vi "GeoData.vi"() -> ()   [LabVIEW 2017] (continued)
County\tH1\n81120\t8023\tAntonito\tCO\tCostilla County\tH1\n81152\t8023\tSan luis\tCO\tCostilla County\tH1\n81151\t8023\tSanford\tCO\tCostilla County\tH1\n81126\t8023\tChama\tCO\tCostilla County\tH1\n81133\t8023\tFort garland\tCO\tCostilla County\tH1\n81123\t8023\tBlanca\tCO\tCostilla County\tH1\n81138\t8023\tJaroso\tCO\tCostilla County\tH1\n81039\t8025\tFowler\tCO\tCrowley County\tH1\n81058\t8025\tManzanola\tCO\tCrowley County\tH1\n81076\t8025\tSugar city\tCO\tCrowley County\tH1\n81034\t8025\tOrdway\tCO\tCrowley County\tH1\n81063\t8025\tOrdway\tCO\tCrowley County\tH1\n81062\t8025\tOlney springs\tCO\tCrowley County\tH1\n81033\t8025\tCrowley\tCO\tCrowley County\tH1\n81252\t8027\tWestcliffe\tCO\tCuster County\tH1\n81223\t8027\tCotopaxi\tCO\tCuster County\tH1\n81253\t8027\tWetmore\tCO\tCuster County\tH1\n81226\t8027\tFlorence\tCO\tCuster County\tH1\n81069\t8027\tRye\tCO\tCuster County\tH1\n81410\t8029\tAustin\tCO\tDelta County\tH1\n81418\t8029\tEckert\tCO\tDelta County\tH1\n81420\t8029\tLazear\tCO\tDelta County\tH1\n81428\t8029\tPaonia\tCO\tDelta County\tH1\n81413\t8029\tCedaredge\tCO\tDelta County\tH1\n81419\t8029\tHotchkiss\tCO\tDelta County\tH1\n81415\t8029\tCrawford\tCO\tDelta County\tH1\n81414\t8029\tCory\tCO\tDelta County\tH1\n81434\t8029\tSomerset\tCO\tDelta County\tH1\n81416\t8029\tDelta\tCO\tDelta County\tH1\n80110\t8031\tEnglewood\tCO\tDenver County\tH6\n80224\t8031\tDenver\tCO\tDenver County\tH6\n80218\t8031\tDenver\tCO\tDenver County\tH6\n80247\t8031\tDenver\tCO\tDenver County\tH6\n80266\t8031\tDenver\tCO\tDenver County\tH6\n80290\t8031\tDenver\tCO\tDenver County\tH6\n80293\t8031\tDenver\tCO\tDenver County\tH6\n80259\t8031\tDenver\tCO\tDenver County\tH6\n80221\t8031\tDenver\tCO\tDenver County\tH6\n80246\t8031\tDenver\tCO\tDenver County\tH6\n80208\t8031\tDenver\tCO\tDenver County\tH6\n80014\t8031\tAurora\tCO\tDenver County\tH6\n80127\t8031\tLittleton\tCO\tDenver County\tH6\n80210\t8031\tDenver\tCO\tDenver County\tH6\n80226\t8031\tDenver\tCO\tDenver County\tH6\n80206\t8031\tDenver\tCO\tDenver County\tH6\n80236\t8031\tDenver\tCO\tDenver County\tH6\n80227\t8031\tDenver\tCO\tDenver County\tH6\n80239\t8031\tDenver\tCO\tDenver County\tH6\n80273\t8031\tDenver\tCO\tDenver County\tH6\n80294\t8031\tDenver\tCO\tDenver County\tH6\n80256\t8031\tDenver\tCO\tDenver County\tH6\n80012\t8031\tAurora\tCO\tDenver County\tH6\n80123\t8031\tLittleton\tCO\tDenver County\tH6\n80111\t8031\tEnglewood\tCO\tDenver County\tH6\n80202\t8031\tDenver\tCO\tDenver County\tH6\n80220\t8031\tDenver\tCO\tDenver County\tH6\n80231\t8031\tDenver\tCO\tDenver County\tH6\n80281\t8031\tDenver\tCO\tDenver County\tH6\n80010\t8031\tAurora\tCO\tDenver County\tH6\n80022\t8031\tCommerce city\tCO\tDenver County\tH6\n80219\t8031\tDenver\tCO\tDenver County\tH6\n80222\t8031\tDenver\tCO\tDenver County\tH6\n80212\t8031\tDenver\tCO\tDenver County\tH6\n80217\t8031\tDenver\tCO\tDenver County\tH6\n80264\t8031\tDenver\tCO\tDenver County\tH6\n80211\t8031\tDenver\tCO\tDenver County\tH6\n80207\t8031\tDenver\tCO\tDenver County\tH6\n80214\t8031\tDenver\tCO\tDenver County\tH6\n80223\t8031\tDenver\tCO\tDenver County\tH6\n80230\t8031\tDenver\tCO\tDenver County\tH6\n80238\t8031\tDenver\tCO\tDenver County\tH6\n80263\t8031\tDenver\tCO\tDenver County\tH6\n80257\t8031\tDenver\tCO\tDenver County\tH6\n80274\t8031\tDenver\tCO\tDenver County\tH6\n80243\t8031\tDenver\tCO\tDenver County\tH6\n80271\t8031\tDenver\tCO\tDenver County\tH6\n80033\t8031\tWheat ridge\tCO\tDenver County\tH6\n80204\t8031\tDenver\tCO\tDenver County\tH6\n80203\t8031\tDenver\tCO\tDenver County\tH6\n80249\t8031\tDenver\tCO\tDenver County\tH6\n80299\t8031\tDenver\tCO\tDenver County\tH6\n80250\t8031\tDenver\tCO\tDenver County\tH6\n80248\t8031\tDenver\tCO\tDenver County\tH6\n80265\t8031\tDenver\tCO\tDenver County\tH6\n80261\t8031\tDenver\tCO\tDenver County\tH6\n80201\t8031\tDenver\tCO\tDenver County\tH6\n80216\t8031\tDenver\tCO\tDenver County\tH6\n80205\t8031\tDenver\tCO\tDenver County\tH6\n80209\t8031\tDenver\tCO\tDenver County\tH6\n80232\t8031\tDenver\tCO\tDenver County\tH6\n80235\t8031\tDenver\tCO\tDenver County\tH6\n80237\t8031\tDenver\tCO\tDenver County\tH6\n80291\t8031\tDenver\tCO\tDenver County\tH6\n81324\t8033\tDove creek\tCO\tDolores County\tH1\n81332\t8033\tRico\tCO\tDolores County\tH1\n81320\t8033\tCahone\tCO\tDolores County\tH1\n80104\t8035\tCastle rock\tCO\tDouglas County\tH1\n80108\t8035\tCastle rock\tCO\tDouglas County\tH1\n80163\t8035\tLittleton\tCO\tDouglas County\tH1\n80112\t8035\tEnglewood\tCO\tDouglas County\tH1\n80125\t8035\tLittleton\tCO\tDouglas County\tH1\n80124\t8035\tLone tree\tCO\tDouglas County\tH1\n80129\t8035\tLittleton\tCO\tDouglas County\tH1\n80126\t8035\tLittleton\tCO\tDouglas County\tH1\n80118\t8035\tLarkspur\tCO\tDouglas County\tH1\n80130\t8035\tLittleton\tCO\tDouglas County\tH1\n80109\t8035\tCastle rock\tCO\tDouglas County\tH1\n80138\t8035\tParker\tCO\tDouglas County\tH1\n80131\t8035\tLouviers\tCO\tDouglas County\tH1\n80016\t8035\tAurora\tCO\tDouglas County\tH1\n80106\t8035\tElbert\tCO\tDouglas County\tH1\n80135\t8035\tSedalia\tCO\tDouglas County\tH1\n80433\t8035\tConifer\tCO\tDouglas County\tH1\n80116\t8035\tFranktown\tCO\tDouglas County\tH1\n80134\t8035\tParker\tCO\tDouglas County\tH1\n81645\t8037\tMinturn\tCO\tEagle County\tH1\n81631\t8037\tEagle\tCO\tEagle County\tH1\n81620\t8037\tAvon\tCO\tEagle County\tH1\n81655\t8037\tWolcott\tCO\tEagle County\tH1\n81649\t8037\tRed cliff\tCO\tEagle County\tH1\n80423\t8037\tBond\tCO\tEagle County\tH1\n81657\t8037\tVail\tCO\tEagle County\tH1\n80498\t8037\tSilverthorne\tCO\tEagle County\tH1\n81621\t8037\tBasalt\tCO\tEagle County\tH1\n81637\t8037\tGypsum\tCO\tEagle County\tH1\n81658\t8037\tVail\tCO\tEagle County\tH1\n80463\t8037\tMc coy\tCO\tEagle County\tH1\n81632\t8037\tEdwards\tCO\tEagle County\tH1\n81623\t8037\tCarbondale\tCO\tEagle County\tH1\n81642\t8037\tMeredith\tCO\tEagle County\tH1\n80426\t8037\tBurns\tCO\tEagle County\tH1\n80832\t8039\tRamah\tCO\tElbert County\tH1\n80105\t8039\tDeer trail\tCO\tElbert County\tH1\n80102\t8039\tBennett\tCO\tElbert County\tH1\n80107\t8039\tElizabeth\tCO\tElbert County\tH1\n80117\t8039\tKiowa\tCO\tElbert County\tH1\n80138\t8039\tParker\tCO\tElbert County\tH1\n80808\t8039\tCalhan\tCO\tElbert County\tH1\n80831\t8039\tPeyton\tCO\tElbert County\tH1\n80101\t8039\tAgate\tCO\tElbert County\tH1\n80106\t8039\tElbert\tCO\tElbert County\tH1\n80116\t8039\tFranktown\tCO\tElbert County\tH1\n80134\t8039\tParker\tCO\tElbert County\tH1\n80833\t8039\tRush\tCO\tElbert County\tH1\n80835\t8039\tSimla\tCO\tElbert County\tH1\n80828\t8039\tLimon\tCO\tElbert County\tH1\n80830\t8039\tMatheson\tCO\tElbert County\tH1\n80903\t8041\tColorado springs\tCO\tEl Paso County\tH1\n80949\t8041\tColorado springs\tCO\tEl Paso County\tH1\n80932\t8041\tColorado springs\tCO\tEl Paso County\tH1\n80901\t8041\tColorado springs\tCO\tEl Paso County\tH1\n80819\t8041\tGreen mountain falls\tCO\tEl Paso County\tH1\n80941\t8041\tColorado springs\tCO\tEl Paso County\tH1\n80917\t8041\tColorado springs\tCO\tEl Paso County\tH1\n80923\t8041\tColorado springs\tCO\tEl Paso County\tH1\n80928\t8041\tColorado springs\tCO\tEl Paso County\tH1\n80933\t8041\tColorado springs\tCO\tEl Paso County\tH1\n80832\t8041\tRamah\tCO\tEl Paso County\tH1\n80938\t8041\tColorado springs\tCO\tEl Paso County\tH1\n80132\t8041\tMonument\tCO\tEl Paso County\tH1\n80921\t8041\tColorado springs\tCO\tEl Paso County\tH1\n80926\t8041\tColorado springs\tCO\tEl Paso County\tH1\n80906\t8041\tColorado springs\tCO\tEl Paso County\tH1\n80907\t8041\tColorado springs\tCO\tEl Paso County\tH1\n80913\t8041\tColorado springs\tCO\tEl Paso County\tH1\n80809\t8041\tCascade\tCO\tEl Paso County\tH1\n80929\t8041\tColorado springs\tCO\tEl Paso County\tH1\n80935\t8041\tColorado springs\tCO\tEl Paso County\tH1\n80841\t8041\tUsaf academy\tCO\tEl Paso County\tH1\n80931\t8041\tColorado springs\tCO\tEl Paso County\tH1\n80942\t8041\tColorado springs\tCO\tEl Paso County\tH1\n80817\t8041\tFountain\tCO\tEl Paso County\tH1\n80920\t8041\tColorado springs\tCO\tEl Paso County\tH1\n80915\t8041\tColorado springs\tCO\tEl Paso County\tH1\n80936\t8041\tColorado springs\tCO\tEl Paso County\tH1\n81008\t8041\tPueblo\tCO\tEl Paso County\tH1\n80133\t8041\tPalmer lake\tCO\tEl Paso County\tH1\n80930\t8041\tColorado springs\tCO\tEl Paso County\tH1\n80977\t8041\tColorado springs\tCO\tEl Paso County\tH1\n80808\t8041\tCalhan\tCO\tEl Paso County\tH1\n80831\t8041\tPeyton\tCO\tEl Paso County\tH1\n80829\t8041\tManitou springs\tCO\tEl Paso County\tH1\n80911\t8041\tColorado springs\tCO\tEl Paso County\tH1\n80908\t8041\tColorado springs\tCO\tEl Paso County\tH1\n80927\t8041\tColorado springs\tCO\tEl Paso County\tH1\n80904\t8041\tColorado springs\tCO\tEl Paso County\tH1\n80924\t8041\tColorado springs\tCO\tEl Paso County\tH1\n80939\t8041\tColorado springs\tCO\tEl Paso County\tH1\n80962\t8041\tColorado springs\tCO\tEl Paso County\tH1\n80934\t8041\tColorado springs\tCO\tEl Paso County\tH1\n80950\t8041\tColorado springs\tCO\tEl Paso County\tH1\n80106\t8041\tElbert\tCO\tEl Paso County\tH1\n80914\t8041\tColorado springs\tCO\tEl Paso County\tH1\n80918\t8041\tColorado springs\tCO\tEl Paso County\tH1\n80919\t8041\tColorado springs\tCO\tEl Paso County\tH1\n80916\t8041\tColorado springs\tCO\tEl Paso County\tH1\n80947\t8041\tColorado springs\tCO\tEl Paso County\tH1\n80946\t8041\tColorado springs\tCO\tEl Paso County\tH1\n80833\t8041\tRush\tCO\tEl Paso County\tH1\n80910\t8041\tColorado springs\tCO\tEl Paso County\tH1\n80909\t8041\tColorado springs\tCO\tEl Paso County\tH1\n80905\t8041\tColorado springs\tCO\tEl Paso County\tH1\n80951\t8041\tColorado springs\tCO\tEl Paso County\tH1\n80840\t8041\tUsaf academy\tCO\tEl Paso County\tH1\n80864\t8041\tYoder\tCO\tEl Paso County\tH1\n80835\t8041\tSimla\tCO\tEl Paso County\tH1\n80912\t8041\tColorado springs\tCO\tEl Paso County\tH1\n80863\t8041\tWoodland park\tCO\tEl Paso County\tH1\n80922\t8041\tColorado springs\tCO\tEl Paso County\tH1\n80902\t8041\tColorado springs\tCO\tEl Paso County\tH1\n80925\t8041\tColorado springs\tCO\tEl Paso County\tH1\n80960\t8041\tColorado springs\tCO\tEl Paso County\tH1\n80970\t8041\tColorado springs\tCO\tEl Paso County\tH1\n80937\t8041\tColorado springs\tCO\tEl Paso County\tH1\n80997\t8041\tColorado springs\tCO\tEl Paso County\tH1\n81240\t8043\tPenrose\tCO\tFremont County\tH1\n81221\t8043\tCoal creek\tCO\tFremont County\tH1\n81232\t8043\tHillside\tCO\tFremont County\tH1\n81252\t8043\tWestcliffe\tCO\tFremont County\tH1\n80926\t8043\tColorado springs\tCO\tFremont County\tH1\n81244\t8043\tRockvale\tCO\tFremont County\tH1\n81212\t8043\tCanon city\tCO\tFremont County\tH1\n81223\t8043\tCotopaxi\tCO\tFremont County\tH1\n81233\t8043\tHoward\tCO\tFremont County\tH1\n81222\t8043\tCoaldale\tCO\tFremont County\tH1\n81290\t8043\tFlorence\tCO\tFremont County\tH1\n81201\t8043\tSalida\tCO\tFremont County\tH1\n81253\t8043\tWetmore\tCO\tFremont County\tH1\n81226\t8043\tFlorence\tCO\tFremont County\tH1\n81215\t8043\tCanon city\tCO\tFremont County\tH1\n80816\t8043\tFlorissant\tCO\tFremont County\tH1\n81641\t8045\tMeeker\tCO\tGarfield County\tH1\n81652\t8045\tSilt\tCO\tGarfield County\tH1\n81647\t8045\tNew castle\tCO\tGarfield County\tH1\n81602\t8045\tGlenwood springs\tCO\tGarfield County\tH1\n81635\t8045\tParachute\tCO\tGarfield County\tH1\n81630\t8045\tDe beque\tCO\tGarfield County\tH1\n81637\t8045\tGypsum\tCO\tGarfield County\tH1\n81601\t8045\tGlenwood springs\tCO\tGarfield County\tH1\n81623\t8045\tCarbondale\tCO\tGarfield County\tH1\n81650\t8045\tRifle\tCO\tGarfield County\tH1\n80422\t8047\tBlack hawk\tCO\tGilpin County\tH1\n80474\t8047\tRollinsville\tCO\tGilpin County\tH1\n80427\t8047\tCentral city\tCO\tGilpin County\tH1\n80403\t8047\tGolden\tCO\tGilpin County\tH1\n80446\t8049\tGranby\tCO\tGrand County\tH1\n80447\t8049\tGrand lake\tCO\tGrand County\tH1\n80442\t8049\tFraser\tCO\tGrand County\tH1\n80482\t8049\tWinter park\tCO\tGrand County\tH1\n80423\t8049\tBond\tCO\tGrand County\tH1\n80498\t8049\tSilverthorne\tCO\tGrand County\tH1\n80459\t8049\tKremmling\tCO\tGrand County\tH1\n80478\t8049\tTabernash\tCO\tGrand County\tH1\n80451\t8049\tHot sulphur springs\tCO\tGrand County\tH1\n80468\t8049\tParshall\tCO\tGrand County\tH1\n81225\t8051\tCrested butte\tCO\tGunnison County\tH1\n81241\t8051\tPitkin\tCO\tGunnison County\tH1\n81428\t8051\tPaonia\tCO\tGunnison County\tH1\n81239\t8051\tParlin\tCO\tGunnison County\tH1\n81230\t8051\tGunnison\tCO\tGunnison County\tH1\n81220\t8051\tCimarron\tCO\tGunnison County\tH1\n81237\t8051\tOhio city\tCO\tGunnison County\tH1\n81210\t8051\tAlmont\tCO\tGunnison County\tH1\n81243\t8051\tPowderhorn\tCO\tGunnison County\tH1\n81434\t8051\tSomerset\tCO\tGunnison County\tH1\n81231\t8051\tGunnison\tCO\tGunnison County\tH1\n81623\t8051\tCarbondale\tCO\tGunnison County\tH1\n81224\t8051\tCrested butte\tCO\tGunnison County\tH1\n81235\t8053\tLake city\tCO\tHinsdale County\tH1\n81147\t8053\tPagosa springs\tCO\tHinsdale County\tH1\n81130\t8053\tCreede\tCO\tHinsdale County\tH1\n81040\t8055\tGardner\tCO\tHuerfano County\tH1\n81089\t8055\tWalsenburg\tCO\tHuerfano County\tH1\n81055\t8055\tLa veta\tCO\tHuerfano County\tH1\n81069\t8055\tRye\tCO\tHuerfano County\tH1\n80430\t8057\tCoalmont\tCO\tJackson County\tH1\n80473\t8057\tRand\tCO\tJackson County\tH1\n80434\t8057\tCowdrey\tCO\tJackson County\tH1\n80480\t8057\tWalden\tCO\tJackson County\tH1\n80439\t8059\tEvergreen\tCO\tJefferson County\tH1\n80454\t8059\tIndian hills\tCO\tJefferson County\tH1\n80004\t8059\tArvada\tCO\tJefferson County\tH1\n80215\t8059\tDenver\tCO\tJefferson County\tH1\n80228\t8059\tDenver\tCO\tJefferson County\tH1\n80401\t8059\tGolden\tCO\tJefferson County\tH1\n80002\t8059\tArvada\tCO\tJefferson County\tH1\n80127\t8059\tLittleton\tCO\tJefferson County\tH1\n80125\t8059\tLittleton\tCO\tJefferson County\tH1\n80226\t8059\tDenver\tCO\tJefferson County\tH1\n80227\t8059\tDenver\tCO\tJefferson County\tH1\n80303\t8059\tBoulder\tCO\tJefferson County\tH1\n80465\t8059\tMorrison\tCO\tJefferson County\tH1\n80162\t8059\tLittleton\tCO\tJefferson County\tH1\n80453\t8059\tIdledale\tCO\tJefferson County\tH1\n80123\t8059\tLittleton\tCO\tJefferson County\tH1\n80437\t8059\tEvergreen\tCO\tJefferson County\tH1\n80006\t8059\tArvada\tCO\tJefferson County\tH1\n80001\t8059\tArvada\tCO\tJefferson County\tH1\n80419\t8059\tGolden\tCO\tJefferson County\tH1\n80003\t8059\tArvada\tCO\tJefferson County\tH1\n80020\t8059\tBroomfield\tCO\tJefferson County\tH1\n80007\t8059\tArvada\tCO\tJefferson County\tH1\n80212\t8059\tDenver\tCO\tJefferson County\tH1\n80021\t8059\tBroomfield\tCO\tJefferson County\tH1\n80031\t8059\tWestminster\tCO\tJefferson County\tH1\n80135\t8059\tSedalia\tCO\tJefferson County\tH1\n80214\t8059\tDenver\tCO\tJefferson County\tH1\n80403\t8059\tGolden\tCO\tJefferson County\tH1\n80433\t8059\tConifer\tCO\tJefferson County\tH1\n80402\t8059\tGolden\tCO\tJefferson County\tH1\n80034\t8059\tWheat ridge\tCO\tJefferson County\tH1\n80457\t8059\tKittredge\tCO\tJefferson County\tH1\n80033\t8059\tWheat ridge\tCO\tJefferson County\tH1\n80128\t8059\tLittleton\tCO\tJefferson County\tH1\n80204\t8059\tDenver\tCO\tJefferson County\tH1\n80421\t8059\tBailey\tCO\tJefferson County\tH1\n80225\t8059\tDenver\tCO\tJefferson County\tH1\n80425\t8059\tBuffalo creek\tCO\tJefferson County\tH1\n80005\t8059\tArvada\tCO\tJefferson County\tH1\n80232\t8059\tDenver\tCO\tJefferson County\tH1\n80235\t8059\tDenver\tCO\tJefferson County\tH1\n80470\t8059\tPine\tCO\tJefferson County\tH1\n81045\t8061\tHaswell\tCO\tKiowa County\tH1\n81092\t8061\tWiley\tCO\tKiowa County\tH1\n81036\t8061\tEads\tCO\tKiowa County\tH1\n81047\t8061\tHolly\tCO\tKiowa County\tH1\n81071\t8061\tSheridan lake\tCO\tKiowa County\tH1\n81021\t8061\tArlington\tCO\tKiowa County\tH1\n80834\t8063\tSeibert\tCO\tKit Carson County\tH1\n80861\t8063\tVona\tCO\tKit Carson County\tH1\n80805\t8063\tBethune\tCO\tKit Carson County\tH1\n80836\t8063\tStratton\tCO\tKit Carson County\tH1\n80807\t8063\tBurlington\tCO\tKit Carson County\tH1\n80815\t8063\tFlagler\tCO\tKit Carson County\tH1\n80461\t8065\tLeadville\tCO\tLake County\tH1\n81251\t8065\tTwin lakes\tCO\tLake County\tH1\n80429\t8065\tClimax\tCO\tLake County\tH1\n81228\t8065\tGranite\tCO\tLake County\tH1\n81326\t8067\tHesperus\tCO\tLa Plata County\tH1\n81137\t8067\tIgnacio\tCO\tLa Plata County\tH1\n81303\t8067\tDurango\tCO\tLa Plata County\tH1\n81302\t8067\tDurango\tCO\tLa Plata County\tH1\n81329\t8067\tMarvel\tCO\tLa Plata County\tH1\n81301\t8067\tDurango\tCO\tLa Plata County\tH1\n81122\t8067\tBayfield\tCO\tLa Plata County\tH1\n81328\t8067\tMancos\tCO\tLa Plata County\tH1\n80549\t8069\tWellington\tCO\tLarimer County\tH1\n80547\t8069\tTimnath\tCO\tLarimer County\tH1\n80525\t8069\tFort collins\tCO\tLarimer County\tH1\n80538\t8069\tLoveland\tCO\tLarimer County\tH1\n80537\t8069\tLoveland\tCO\tLarimer County\tH1\n80553\t8069\tFort collins\tCO\tLarimer County\tH1\n80513\t8069\tBerthoud\tCO\tLarimer County\tH1\n80517\t8069\tEstes park\tCO\tLarimer County\tH1\n80521\t8069\tFort collins\tCO\tLarimer County\tH1\n80430\t8069\tCoalmont\tCO\tLarimer County\tH1\n80512\t8069\tBellvue\tCO\tLarimer County\tH1\n80510\t8069\tAllenspark\tCO\tLarimer County\tH1\n80532\t8069\tGlen haven\tCO\tLarimer County\tH1\n80511\t8069\tEstes park\tCO\tLarimer County\tH1\n80535\t8069\tLaporte\tCO\tLarimer County\tH1\n80527\t8069\tFort collins\tCO\tLarimer County\tH1\n80503\t8069\tLongmont\tCO\tLarimer County\tH1\n80541\t8069\tMasonville\tCO\tLarimer County\tH1\n80528\t8069\tFort collins\tCO\tLarimer County\tH1\n80534\t8069\tJohnstown\tCO\tLarimer County\tH1\n80545\t8069\tRed feather lakes\tCO\tLarimer County\tH1\n80524\t8069\tFort collins\tCO\tLarimer County\tH1\n80536\t8069\tLivermore\tCO\tLarimer County\tH1\n80522\t8069\tFort collins\tCO\tLarimer County\tH1\n80526\t8069\tFort collins\tCO\tLarimer County\tH1\n80550\t8069\tWindsor\tCO\tLarimer County\tH1\n80504\t8069\tLongmont\tCO\tLarimer County\tH1\n80515\t8069\tDrake\tCO\tLarimer County\tH1\n80612\t8069\tCarr\tCO\tLarimer County\tH1\n80540\t8069\tLyons\tCO\tLarimer County\tH1\n80523\t8069\tFort collins\tCO\tLarimer County\tH1\n80539\t8069\tLoveland\tCO\tLarimer County\tH1\n81039\t8071\tFowler\tCO\tLas Animas County\tH1\n81046\t8071\tHoehne\tCO\tLas Animas County\tH1\n81089\t8071\tWalsenburg\tCO\tLas Animas County\tH1\n81020\t8071\tAguilar\tCO\tLas Animas County\tH1\n81081\t8071\tTrinchera\tCO\tLas Animas County\tH1\n81091\t8071\tWeston\tCO\tLas Animas County\tH1\n81024\t8071\tBoncarbo\tCO\tLas Animas County\tH1\n81082\t8071\tTrinidad\tCO\tLas Animas County\tH1\n81049\t8071\tKim\tCO\tLas Animas County\tH1\n81027\t8071\tBranson\tCO\tLas Animas County\tH1\n81054\t8071\tLas animas\tCO\tLas Animas County\tH1\n81059\t8071\tModel\tCO\tLas Animas County\tH1\n81064\t8071\tPritchett\tCO\tLas Animas County\tH1\n81076\t8073\tSugar city\tCO\tLincoln County\tH1\n80826\t8073\tLimon\tCO\tLincoln County\tH1\n80832\t8073\tRamah\tCO\tLincoln County\tH1\n81045\t8073\tHaswell\tCO\tLincoln County\tH1\n80821\t8073\tHugo\tCO\tLincoln County\tH1\n81063\t8073\tOrdway\tCO\tLincoln County\tH1\n80804\t8073\tArriba\tCO\tLincoln County\tH1\n80833\t8073\tRush\tCO\tLincoln County\tH1\n80815\t8073\tFlagler\tCO\tLincoln County\tH1\n81021\t8073\tArlington\tCO\tLincoln County\tH1\n80828\t8073\tLimon\tCO\tLincoln County\tH1\n80823\t8073\tKarval\tCO\tLincoln County\tH1\n80818\t8073\tGenoa\tCO\tLincoln County\tH1\n80741\t8075\tMerino\tCO\tLogan County\tH1\n80726\t8075\tCrook\tCO\tLogan County\tH1\n80751\t8075\tSterling\tCO\tLogan County\tH1\n80731\t8075\tHaxtun\tCO\tLogan County\tH1\n80747\t8075\tPeetz\tCO\tLogan County\tH1\n80745\t8075\tPadroni\tCO\tLogan County\tH1\n80736\t8075\tIliff\tCO\tLogan County\tH1\n80728\t8075\tFleming\tCO\tLogan County\tH1\n80722\t8075\tAtwood\tCO\tLogan County\tH1\n81523\t8077\tGlade park\tCO\tMesa County\tH1\n81504\t8077\tGrand junction\tCO\tMesa County\tH1\n81521\t8077\tFruita\tCO\tMesa County\tH1\n81507\t8077\tGrand junction\tCO\tMesa County\tH1\n81502\t8077\tGrand junction\tCO\tMesa County\tH1\n81635\t8077\tParachute\tCO\tMesa County\tH1\n81520\t8077\tClifton\tCO\tMesa County\tH1\n81505\t8077\tGrand junction\tCO\tMesa County\tH1\n81524\t8077\tLoma\tCO\tMesa County\tH1\n81501\t8077\tGrand junction\tCO\tMesa County\tH1\n81527\t8077\tWhitewater\tCO\tMesa County\tH1\n81525\t8077\tMack\tCO\tMesa County\tH1\n81630\t8077\tDe beque\tCO\tMesa County\tH1\n81522\t8077\tGateway\tCO\tMesa County\tH1\n81503\t8077\tGrand junction\tCO\tMesa County\tH1\n81506\t8077\tGrand junction\tCO\tMesa County\tH1\n81646\t8077\tMolina\tCO\tMesa County\tH1\n81526\t8077\tPalisade\tCO\tMesa County\tH1\n81624\t8077\tCollbran\tCO\tMesa County\tH1\n81643\t8077\tMesa\tCO\tMesa County\tH1\n81154\t8079\tSouth fork\tCO\tMineral County\tH1\n81130\t8079\tCreede\tCO\tMineral County\tH1\n81638\t8081\tHamilton\tCO\tMoffat County\tH1\n81641\t8081\tMeeker\tCO\tMoffat County\tH1\n81610\t8081\tDinosaur\tCO\tMoffat County\tH1\n81653\t8081\tSlater\tCO\tMoffat County\tH1\n81633\t8081\tDinosaur\tCO\tMoffat County\tH1\n81640\t8081\tMaybell\tCO\tMoffat County\tH1\n81625\t8081\tCraig\tCO\tMoffat County\tH1\n81335\t8083\tYellow jacket\tCO\tMontezuma County\tH1\n81330\t8083\tMesa verde national park\tCO\tMontezuma County\tH1\n81323\t8083\tDolores\tCO\tMontezuma County\tH1\n81321\t8083\tCortez\tCO\tMontezuma County\tH1\n81328\t8083\tMancos\tCO\tMontezuma County\tH1\n81327\t8083\tLewis\tCO\tMontezuma County\tH1\n81331\t8083\tPleasant view\tCO\tMontezuma County\tH1\n81334\t8083\tTowaoc\tCO\tMontezuma County\tH1\n81402\t8085\tMontrose\tCO\tMontrose County\tH1\n81424\t8085\tNucla\tCO\tMontrose County\tH1\n81220\t8085\tCimarron\tCO\tMontrose County\tH1\n81429\t8085\tParadox\tCO\tMontrose County\tH1\n81403\t8085\tMontrose\tCO\tMontrose County\tH1\n81425\t8085\tOlathe\tCO\tMontrose County\tH1\n81415\t8085\tCrawford\tCO\tMontrose County\tH1\n81401\t8085\tMontrose\tCO\tMontrose County\tH1\n81411\t8085\tBedrock\tCO\tMontrose County\tH1\n81416\t8085\tDelta\tCO\tMontrose County\tH1\n81431\t8085\tRedvale\tCO\tMontrose County\tH1\n81422\t8085\tNaturita\tCO\tMontrose County\tH1\n80701\t8087\tFort morgan\tCO\tMorgan County\tH1\n80654\t8087\tWiggins\tCO\tMorgan County\tH1\n80741\t8087\tMerino\tCO\tMorgan County\tH1\n80653\t8087\tWeldona\tCO\tMorgan County\tH1\n80705\t8087\tLog lane village\tCO\tMorgan County\tH1\n80754\t8087\tStoneham\tCO\tMorgan County\tH1\n80649\t8087\tOrchard\tCO\tMorgan County\tH1\n80733\t8087\tHillrose\tCO\tMorgan County\tH1\n80750\t8087\tSnyder\tCO\tMorgan County\tH1\n80723\t8087\tBrush\tCO\tMorgan County\tH1\n80742\t8087\tNew raymer\tCO\tMorgan County\tH1\n81039\t8089\tFowler\tCO\tOtero County\tH1\n81058\t8089\tManzanola\tCO\tOtero County\tH1\n81050\t8089\tLa junta\tCO\tOtero County\tH1\n81030\t8089\tCheraw\tCO\tOtero County\tH1\n81067\t8089\tRocky ford\tCO\tOtero County\tH1\n81024\t8089\tBoncarbo\tCO\tOtero County\tH1\n81082\t8089\tTrinidad\tCO\tOtero County\tH1\n81077\t8089\tSwink\tCO\tOtero County\tH1\n81059\t8089\tModel\tCO\tOtero County\tH1\n81432\t8091\tRidgway\tCO\tOuray County\tH1\n81403\t8091\tMontrose\tCO\tOuray County\tH1\n81427\t8091\tOuray\tCO\tOuray County\tH1\n80827\t8093\tLake george\tCO\tPark County\tH1\n80420\t8093\tAlma\tCO\tPark County\tH1\n80432\t8093\tComo\tCO\tPark County\tH1\n80475\t8093\tShawnee\tCO\tPark County\tH1\n80448\t8093\tGrant\tCO\tPark County\tH1\n80456\t8093\tJefferson\tCO\tPark County\tH1\n80440\t8093\tFairplay\tCO\tPark County\tH1\n80421\t8093\tBailey\tCO\tPark County\tH1\n80816\t8093\tFlorissant\tCO\tPark County\tH1\n80820\t8093\tGuffey\tCO\tPark County\tH1\n80470\t8093\tPine\tCO\tPark County\tH1\n80449\t8093\tHartsel\tCO\tPark County\tH1\n80731\t8095\tHaxtun\tCO\tPhillips County\tH1\n80721\t8095\tAmherst\tCO\tPhillips County\tH1\n80734\t8095\tHolyoke\tCO\tPhillips County\tH1\n80744\t8095\tOvid\tCO\tPhillips County\tH1\n80746\t8095\tPaoli\tCO\tPhillips County\tH1\n81654\t8097\tSnowmass\tCO\tPitkin County\tH1\n81611\t8097\tAspen\tCO\tPitkin County\tH1\n81615\t8097\tSnowmass village\tCO\tPitkin County\tH1\n81621\t8097\tBasalt\tCO\tPitkin County\tH1\n81656\t8097\tWoody creek\tCO\tPitkin County\tH1\n81612\t8097\tAspen\tCO\tPitkin County\tH1\n81623\t8097\tCarbondale\tCO\tPitkin County\tH1\n81642\t8097\tMeredith\tCO\tPitkin County\tH1\n81052\t8099\tLamar\tCO\tProwers County\tH1\n81092\t8099\tWiley\tCO\tProwers County\tH1\n81043\t8099\tHartman\tCO\tProwers County\tH1\n81090\t8099\tWalsh\tCO\tProwers County\tH1\n81047\t8099\tHolly\tCO\tProwers County\tH1\n81041\t8099\tGranada\tCO\tProwers County\tH1\n81039\t8101\tFowler\tCO\tPueblo County\tH1\n81002\t8101\tPueblo\tCO\tPueblo County\tH1\n81010\t8101\tPueblo\tCO\tPueblo County\tH1\n81007\t8101\tPueblo\tCO\tPueblo County\tH1\n81009\t8101\tPueblo\tCO\tPueblo County\tH1\n80817\t8101\tFountain\tCO\tPueblo County\tH1\n81004\t8101\tPueblo\tCO\tPueblo County\tH1\n81008\t8101\tPueblo\tCO\tPueblo County\tH1\n81025\t8101\tBoone\tCO\tPueblo County\tH1\n81062\t8101\tOlney springs\tCO\tPueblo County\tH1\n81001\t8101\tPueblo\tCO\tPueblo County\tH1\n81023\t8101\tBeulah\tCO\tPueblo County\tH1\n81253\t8101\tWetmore\tCO\tPueblo County\tH1\n81006\t8101\tPueblo\tCO\tPueblo County\tH1\n81011\t8101\tPueblo\tCO\tPueblo County\tH1\n81012\t8101\tPueblo\tCO\tPueblo County\tH1\n81022\t8101\tAvondale\tCO\tPueblo County\tH1\n81069\t8101\tRye\tCO\tPueblo County\tH1\n81005\t8101\tPueblo\tCO\tPueblo County\tH1\n81003\t8101\tPueblo\tCO\tPueblo County\tH1\n81019\t8101\tColorado city\tCO\tPueblo County\tH1\n81638\t8103\tHamilton\tCO\tRio Blanco County\tH1\n81641\t8103\tMeeker\tCO\tRio Blanco County\tH1\n81648\t8103\tRangely\tCO\tRio Blanco County\tH1\n81650\t8103\tRifle\tCO\tRio Blanco County\tH1\n81135\t8105\tHomelake\tCO\tRio Grande County\tH1\n81101\t8105\tAlamosa\tCO\tRio Grande County\tH1\n81132\t8105\tDel norte\tCO\tRio Grande County\tH1\n81125\t8105\tCenter\tCO\tRio Grande County\tH1\n81140\t8105\tLa jara\tCO\tRio Grande County\tH1\n81154\t8105\tSouth fork\tCO\tRio Grande County\tH1\n81144\t8105\tMonte vista\tCO\tRio Grande County\tH1\n81638\t8107\tHamilton\tCO\tRoutt County\tH1\n80483\t8107\tYampa\tCO\tRoutt County\tH1\n80467\t8107\tOak creek\tCO\tRoutt County\tH1\n81639\t8107\tHayden\tCO\tRoutt County\tH1\n80479\t8107\tToponas\tCO\tRoutt County\tH1\n80469\t8107\tPhippsburg\tCO\tRoutt County\tH1\n80487\t8107\tSteamboat springs\tCO\tRoutt County\tH1\n80463\t8107\tMc coy\tCO\tRoutt County\tH1\n80477\t8107\tSteamboat springs\tCO\tRoutt County\tH1\n80428\t8107\tClark\tCO\tRoutt County\tH1\n81155\t8109\tVilla grove\tCO\tSaguache County\tH1\n81149\t8109\tSaguache\tCO\tSaguache County\tH1\n81230\t8109\tGunnison\tCO\tSaguache County\tH1\n81143\t8109\tMoffat\tCO\tSaguache County\tH1\n81132\t8109\tDel norte\tCO\tSaguache County\tH1\n81248\t8109\tSargents\tCO\tSaguache County\tH1\n81125\t8109\tCenter\tCO\tSaguache County\tH1\n81136\t8109\tHooper\tCO\tSaguache County\tH1\n81131\t8109\tCrestone\tCO\tSaguache County\tH1\n81432\t8111\tRidgway\tCO\tSan Juan County\tH1\n81301\t8111\tDurango\tCO\tSan Juan County\tH1\n81433\t8111\tSilverton\tCO\tSan Juan County\tH1\n81435\t8113\tTelluride\tCO\tSan Miguel County\tH1\n81432\t8113\tRidgway\tCO\tSan Miguel County\tH1\n81426\t8113\tOphir\tCO\tSan Miguel County\tH1\n81423\t8113\tNorwood\tCO\tSan Miguel County\tH1\n81325\t8113\tEgnar\tCO\tSan Miguel County\tH1\n81430\t8113\tPlacerville\tCO\tSan Miguel County\tH1\n80721\t8115\tAmherst\tCO\tSedgwick County\tH1\n80737\t8115\tJulesburg\tCO\tSedgwick County\tH1\n80749\t8115\tSedgwick\tCO\tSedgwick County\tH1\n80744\t8115\tOvid\tCO\tSedgwick County\tH1\n80443\t8117\tFrisco\tCO\tSummit County\tH1\n80424\t8117\tBreckenridge\tCO\tSummit County\tH1\n80435\t8117\tDillon\tCO\tSummit County\tH1\n80497\t8117\tSilverthorne\tCO\tSummit County\tH1\n80498\t8117\tSilverthorne\tCO\tSummit County\tH1\n80813\t8119\tCripple creek\tCO\tTeller County\tH1\n80827\t8119\tLake george\tCO\tTeller County\tH1\n80814\t8119\tDivide\tCO\tTeller County\tH1\n80906\t8119\tColorado springs\tCO\tTeller County\tH1\n80866\t8119\tWoodland park\tCO\tTeller County\tH1\n80860\t8119\tVictor\tCO\tTeller County\tH1\n80135\t8119\tSedalia\tCO\tTeller County\tH1\n80816\t8119\tFlorissant\tCO\tTeller County\tH1\n80863\t8119\tWoodland park\tCO\tTeller County\tH1\n80741\t8121\tMerino\tCO\tWashington County\tH1\n80834\t8121\tSeibert\tCO\tWashington County\tH1\n80759\t8121\tYuma\tCO\tWashington County\tH1\n80743\t8121\tOtis\tCO\tWashington County\tH1\n80812\t8121\tCope\tCO\tWashington County\tH1\n80801\t8121\tAnton\tCO\tWashington County\tH1\n80733\t8121\tHillrose\tCO\tWashington County\tH1\n80757\t8121\tWoodrow\tCO\tWashington County\tH1\n80723\t8121\tBrush\tCO\tWashington County\tH1\n80720\t8121\tAkron\tCO\tWashington County\tH1\n80818\t8121\tGenoa\tCO\tWashington County\tH1\n80740\t8121\tLindon\tCO\tWashington County\tH1\n80642\t8123\tHudson\tCO\tWeld County\tH1\n80549\t8123\tWellington\tCO\tWeld County\tH1\n80654\t8123\tWiggins\tCO\tWeld County\tH1\n80729\t8123\tGrover\tCO\tWeld County\tH1\n80741\t8123\tMerino\tCO\tWeld County\tH1\n80520\t8123\tFirestone\tCO\tWeld County\tH1\n80646\t8123\tLucerne\tCO\tWeld County\tH1\n80537\t8123\tLoveland\tCO\tWeld County\tH1\n80732\t8123\tHereford\tCO\tWeld County\tH1\n80615\t8123\tEaton\tCO\tWeld County\tH1\n80513\t8123\tBerthoud\tCO\tWeld County\tH1\n80645\t8123\tLa salle\tCO\tWeld County\tH1\n80648\t8123\tNunn\tCO\tWeld County\tH1\n80754\t8123\tStoneham\tCO\tWeld County\tH1\n80634\t8123\tGreeley\tCO\tWeld County\tH1\n80644\t8123\tKersey\tCO\tWeld County\tH1\n80632\t8123\tGreeley\tCO\tWeld County\tH1\n80543\t8123\tMilliken\tCO\tWeld County\tH1\n80516\t8123\tErie\tCO\tWeld County\tH1\n80649\t8123\tOrchard\tCO\tWeld County\tH1\n80624\t8123\tGill\tCO\tWeld County\tH1\n80620\t8123\tEvans\tCO\tWeld County\tH1\n80745\t8123\tPadroni\tCO\tWeld County\tH1\n80611\t8123\tBriggsdale\tCO\tWeld County\tH1\n80633\t8123\tGreeley\tCO\tWeld County\tH1\n80631\t8123\tGreeley\tCO\tWeld County\tH1\n80534\t8123\tJohnstown\tCO\tWeld County\tH1\n80621\t8123\tFort lupton\tCO\tWeld County\tH1\n80643\t8123\tKeenesburg\tCO\tWeld County\tH1\n80524\t8123\tFort collins\tCO\tWeld County\tH1\n80542\t8123\tMead\tCO\tWeld County\tH1\n80651\t8123\tPlatteville\tCO\tWeld County\tH1\n80639\t8123\tGreeley\tCO\tWeld County\tH1\n80652\t8123\tRoggen\tCO\tWeld County\tH1\n80550\t8123\tWindsor\tCO\tWeld County\tH1\n80504\t8123\tLongmont\tCO\tWeld County\tH1\n80514\t8123\tDacono\tCO\tWeld County\tH1\n80530\t8123\tFrederick\tCO\tWeld County\tH1\n80612\t8123\tCarr\tCO\tWeld County\tH1\n80650\t8123\tPierce\tCO\tWeld County\tH1\n80546\t8123\tSeverance\tCO\tWeld County\tH1\n80622\t8123\tGaleton\tCO\tWeld County\tH1\n80638\t8123\tGreeley\tCO\tWeld County\tH1\n80551\t8123\tWindsor\tCO\tWeld County\tH1\n80603\t8123\tBrighton\tCO\tWeld County\tH1\n80742\t8123\tNew raymer\tCO\tWeld County\tH1\n80610\t8123\tAult\tCO\tWeld County\tH1\n80623\t8123\tGilcrest\tCO\tWeld County\tH1\n80758\t8125\tWray\tCO\tYuma County\tH1\n80822\t8125\tJoes\tCO\tYuma County\tH1\n80727\t8125\tEckley\tCO\tYuma County\tH1\n80824\t8125\tKirk\tCO\tYuma County\tH1\n80731\t8125\tHaxtun\tCO\tYuma County\tH1\n80755\t8125\tVernon\tCO\tYuma County\tH1\n80759\t8125\tYuma\tCO\tYuma County\tH1\n80812\t8125\tCope\tCO\tYuma County\tH1\n80734\t8125\tHolyoke\tCO\tYuma County\tH1\n80735\t8125\tIdalia\tCO\tYuma County\tH1\n80807\t8125\tBurlington\tCO\tYuma County\tH1\n6484\t9001\tShelton\tCT\tFairfield County\tH4\n6608\t9001\tBridgeport\tCT\tFairfield County\tH4\n6824\t9001\tFairfield\tCT\tFairfield County\tH4\n6807\t9001\tCos cob\tCT\tFairfield County\tH4\n6830\t9001\tGreenwich\tCT\tFairfield County\tH4\n6903\t9001\tStamford\tCT\tFairfield County\tH4\n6910\t9001\tStamford\tCT\tFairfield County\tH4\n6602\t9001\tBridgeport\tCT\tFairfield County\tH4\n6801\t9001\tBethel\tCT\tFairfield County\tH4\n6813\t9001\tDanbury\tCT\tFairfield County\tH4\n6825\t9001\tFairfield\tCT\tFairfield County\tH4\n6851\t9001\tNorwalk\tCT\tFairfield County\tH4\n6902\t9001\tStamford\tCT\tFairfield County\tH4\n6904\t9001\tStamford\tCT\tFairfield County\tH4\n6890\t9001\tSouthport\tCT\tFairfield County\tH4\n6901\t9001\tStamford\tCT\tFairfield County\tH4\n6673\t9001\tBridgeport\tCT\tFairfield County\tH4\n6828\t9001\tFairfield\tCT\tFairfield County\tH4\n6875\t9001\tRedding center\tCT\tFairfield County\tH4\n6470\t9001\tNewtown\tCT\tFairfield County\tH4\n6811\t9001\tDanbury\tCT\tFairfield County\tH4\n6810\t9001\tDanbury\tCT\tFairfield County\tH4\n6784\t9001\tSherman\tCT\tFairfield County\tH4\n6853\t9001\tNorwalk\tCT\tFairfield County\tH4\n6836\t9001\tGreenwich\tCT\tFairfield County\tH4\n6911\t9001\tStamford\tCT\tFairfield County\tH4\n6926\t9001\tStamford\tCT\tFairfield County\tH4\n6856\t9001\tNorwalk\tCT\tFairfield County\tH4\n6858\t9001\tNorwalk\tCT\tFairfield County\tH4\n6912\t9001\tStamford\tCT\tFairfield County\tH4\n6888\t9001\tWestport\tCT\tFairfield County\tH4\n6418\t9001\tDerby\tCT\tFairfield County\tH4\n6468\t9001\tMonroe\tCT\tFairfield County\tH4\n6605\t9001\tBridgeport\tCT\tFairfield County\tH4\n6610\t9001\tBridgeport\tCT\tFairfield County\tH4\n6606\t9001\tBridgeport\tCT\tFairfield County\tH4\n6804\t9001\tBrookfield\tCT\tFairfield County\tH4\n6870\t9001\tOld greenwich\tCT\tFairfield County\tH4\n6907\t9001\tStamford\tCT\tFairfield County\tH4\n6883\t9001\tWeston\tCT\tFairfield County\tH4\n6440\t9001\tHawleyville\tCT\tFairfield County\tH4\n6604\t9001\tBridgeport\tCT\tFairfield County\tH4\n6820\t9001\tDarien\tCT\tFairfield County\tH4\n6831\t9001\tGreenwich\tCT\tFairfield County\tH4\n6855\t9001\tNorwalk\tCT\tFairfield County\tH4\n6897\t9001\tWilton\tCT\tFairfield County\tH4\n6829\t9001\tGeorgetown\tCT\tFairfield County\tH4\n6881\t9001\tWestport\tCT\tFairfield County\tH4\n6927\t9001\tStamford\tCT\tFairfield County\tH4\n6482\t9001\tSandy hook\tCT\tFairfield County\tH4\n6612\t9001\tEaston\tCT\tFairfield County\tH4\n6614\t9001\tStratford\tCT\tFairfield County\tH4\n6615\t9001\tStratford\tCT\tFairfield County\tH4\n6607\t9001\tBridgeport\tCT\tFairfield County\tH4\n6776\t9001\tNew milford\tCT\tFairfield County\tH4\n6812\t9001\tNew fairfield\tCT\tFairfield County\tH4\n6840\t9001\tNew canaan\tCT\tFairfield County\tH4\n6854\t9001\tNorwalk\tCT\tFairfield County\tH4\n6850\t9001\tNorwalk\tCT\tFairfield County\tH4\n6905\t9001\tStamford\tCT\tFairfield County\tH4\n6896\t9001\tRedding\tCT\tFairfield County\tH4\n6404\t9001\tBotsford\tCT\tFairfield County\tH4\n6699\t9001\tBridgeport\tCT\tFairfield County\tH4\n6852\t9001\tNorwalk\tCT\tFairfield County\tH4\n6876\t9001\tRedding ridge\tCT\tFairfield County\tH4\n6611\t9001\tTrumbull\tCT\tFairfield County\tH4\n6880\t9001\tWestport\tCT\tFairfield County\tH4\n6877\t9001\tRidgefield\tCT\tFairfield County\tH4\n6878\t9001\tRiverside\tCT\tFairfield County\tH4\n6906\t9001\tStamford\tCT\tFairfield County\tH4\n6838\t9001\tGreens farms\tCT\tFairfield County\tH4\n6601\t9001\tBridgeport\tCT\tFairfield County\tH4\n6491\t9001\tStevenson\tCT\tFairfield County\tH4\n6040\t9003\tManchester\tCT\tHartford County\tH4\n6016\t9003\tBroad brook\tCT\tHartford County\tH4\n6035\t9003\tGranby\tCT\tHartford County\tH4\n6013\t9003\tBurlington\tCT\tHartford County\tH4\n6066\t9003\tVernon rockville\tCT\tHartford County\tH4\n6073\t9003\tSouth glastonbury\tCT\tHartford County\tH4\n6093\t9003\tWest suffield\tCT\tHartford County\tH4\n6786\t9003\tTerryville\tCT\tHartford County\tH4\n6131\t9003\tNewington\tCT\tHartford County\tH4\n6115\t9003\tHartford\tCT\tHartford County\tH4\n6147\t9003\tHartford\tCT\tHartford County\tH4\n6154\t9003\tHartford\tCT\tHartford County\tH4\n6001\t9003\tAvon\tCT\tHartford County\tH4\n6026\t9003\tEast granby\tCT\tHartford County\tH4\n6108\t9003\tEast hartford\tCT\tHartford County\tH4\n6489\t9003\tSouthington\tCT\tHartford County\tH4\n6045\t9003\tManchester\tCT\tHartford County\tH4\n6092\t9003\tWest simsbury\tCT\tHartford County\tH4\n6089\t9003\tWeatogue\tCT\tHartford County\tH4\n6156\t9003\tHartford\tCT\tHartford County\tH4\n6101\t9003\tHartford\tCT\tHartford County\tH4\n6052\t9003\tNew britain\tCT\tHartford County\tH4\n6088\t9003\tEast windsor\tCT\tHartford County\tH4\n6114\t9003\tHartford\tCT\tHartford County\tH4\n6023\t9003\tEast berlin\tCT\tHartford County\tH4\n6011\t9003\tBristol\tCT\tHartford County\tH4\n6090\t9003\tWest granby\tCT\tHartford County\tH4\n6138\t9003\tEast hartford\tCT\tHartford County\tH4\n6144\t9003\tHartford\tCT\tHartford County\tH4\n6146\t9003\tHartford\tCT\tHartford County\tH4\n6141\t9003\tHartford\tCT\tHartford County\tH4\n6143\t9003\tHartford\tCT\tHartford County\tH4\n6145\t9003\tHartford\tCT\tHartford County\tH4\n6030\t9003\tFarmington\tCT\tHartford County\tH4\n6167\t9003\tHartford\tCT\tHartford County\tH4\n6152\t9003\tHartford\tCT\tHartford County\tH4\n6467\t9003\tMilldale\tCT\tHartford County\tH4\n6002\t9003\tBloomfield\tCT\tHartford County\tH4\n6019\t9003\tCanton\tCT\tHartford County\tH4\n6078\t9003\tSuffield\tCT\tHartford County\tH4\n6062\t9003\tPlainville\tCT\tHartford County\tH4\n6067\t9003\tRocky hill\tCT\tHartford County\tH4\n6070\t9003\tSimsbury\tCT\tHartford County\tH4\n6053\t9003\tNew britain\tCT\tHartford County\tH4\n6109\t9003\tWethersfield\tCT\tHartford County\tH4\n6103\t9003\tHartford\tCT\tHartford County\tH4\n6444\t9003\tMarion\tCT\tHartford County\tH4\n6791\t9003\tHarwinton\tCT\tHartford County\tH4\n6034\t9003\tFarmington\tCT\tHartford County\tH4\n6083\t9003\tEnfield\tCT\tHartford County\tH4\n6155\t9003\tHartford\tCT\tHartford County\tH4\n6006\t9003\tWindsor\tCT\tHartford County\tH4\n6028\t9003\tEast windsor hill\tCT\tHartford County\tH4\n6041\t9003\tManchester\tCT\tHartford County\tH4\n6051\t9003\tNew britain\tCT\tHartford County\tH4\n6037\t9003\tBerlin\tCT\tHartford County\tH4\n6020\t9003\tCanton center\tCT\tHartford County\tH4\n6027\t9003\tEast hartland\tCT\tHartford County\tH4\n6074\t9003\tSouth windsor\tCT\tHartford County\tH4\n6060\t9003\tNorth granby\tCT\tHartford County\tH4\n6111\t9003\tNewington\tCT\tHartford County\tH4\n6112\t9003\tHartford\tCT\tHartford County\tH4\n6117\t9003\tWest hartford\tCT\tHartford County\tH4\n6119\t9003\tWest hartford\tCT\tHartford County\tH4\n6126\t9003\tHartford\tCT\tHartford County\tH4\n6451\t9003\tMeriden\tCT\tHartford County\tH4\n6064\t9003\tPoquonock\tCT\tHartford County\tH4\n6065\t9003\tRiverton\tCT\tHartford County\tH4\n6127\t9003\tWest hartford\tCT\tHartford County\tH4\n6022\t9003\tCollinsville\tCT\tHartford County\tH4\n6153\t9003\tHartford\tCT\tHartford County\tH4\n6010\t9003\tBristol\tCT\tHartford County\tH4\n6032\t9003\tFarmington\tCT\tHartford County\tH4\n6033\t9003\tGlastonbury\tCT\tHartford County\tH4\n6042\t9003\tManchester\tCT\tHartford County\tH4\n6043\t9003\tBolton\tCT\tHartford County\tH4\n6082\t9003\tEnfield\tCT\tHartford County\tH4\n6071\t9003\tSomers\tCT\tHartford County\tH4\n6096\t9003\tWindsor locks\tCT\tHartford County\tH4\n6110\t9003\tWest hartford\tCT\tHartford County\tH4\n6095\t9003\tWindsor\tCT\tHartford County\tH4\n6118\t9003\tEast hartford\tCT\tHartford County\tH4\n6479\t9003\tPlantsville\tCT\tHartford County\tH4\n6091\t9003\tWest hartland\tCT\tHartford County\tH4\n6137\t9003\tWest hartford\tCT\tHartford County\tH4\n6123\t9003\tHartford\tCT\tHartford County\tH4\n6142\t9003\tHartford\tCT\tHartford County\tH4\n6102\t9003\tHartford\tCT\tHartford County\tH4\n6025\t9003\tEast glastonbury\tCT\tHartford County\tH4\n6080\t9003\tSuffield\tCT\tHartford County\tH4\n6105\t9003\tHartford\tCT\tHartford County\tH4\n6106\t9003\tHartford\tCT\tHartford County\tH4\n6107\t9003\tWest hartford\tCT\tHartford County\tH4\n6085\t9003\tUnionville\tCT\tHartford County\tH4\n6133\t9003\tWest hartford\tCT\tHartford County\tH4\n6129\t9003\tWethersfield\tCT\tHartford County\tH4\n6081\t9003\tTariffville\tCT\tHartford County\tH4\n6128\t9003\tEast hartford\tCT\tHartford County\tH4\n6161\t9003\tHartford\tCT\tHartford County\tH4\n6050\t9003\tNew britain\tCT\tHartford County\tH4\n6120\t9003\tHartford\tCT\tHartford County\tH4\n6134\t9003\tHartford\tCT\tHartford County\tH4\n6447\t9003\tMarlborough\tCT\tHartford County\tH4\n6160\t9003\tHartford\tCT\tHartford County\tH4\n6132\t9003\tHartford\tCT\tHartford County\tH4\n6183\t9003\tHartford\tCT\tHartford County\tH4\n6199\t9003\tHartford\tCT\tHartford County\tH4\n6021\t9005\tColebrook\tCT\tLitchfield County\tH4\n6057\t9005\tNew hartford\tCT\tLitchfield 
